vi "Alarms FP FGV.vi"(6 "FP Open in":bool, 7 "Function":enum16{"Read", "Write", "Clear"}(ring)) -> (2 "FP Open out":bool)   [LabVIEW 2020]
panel:
  out "error out":errorcluster
  in  "error in":errorcluster
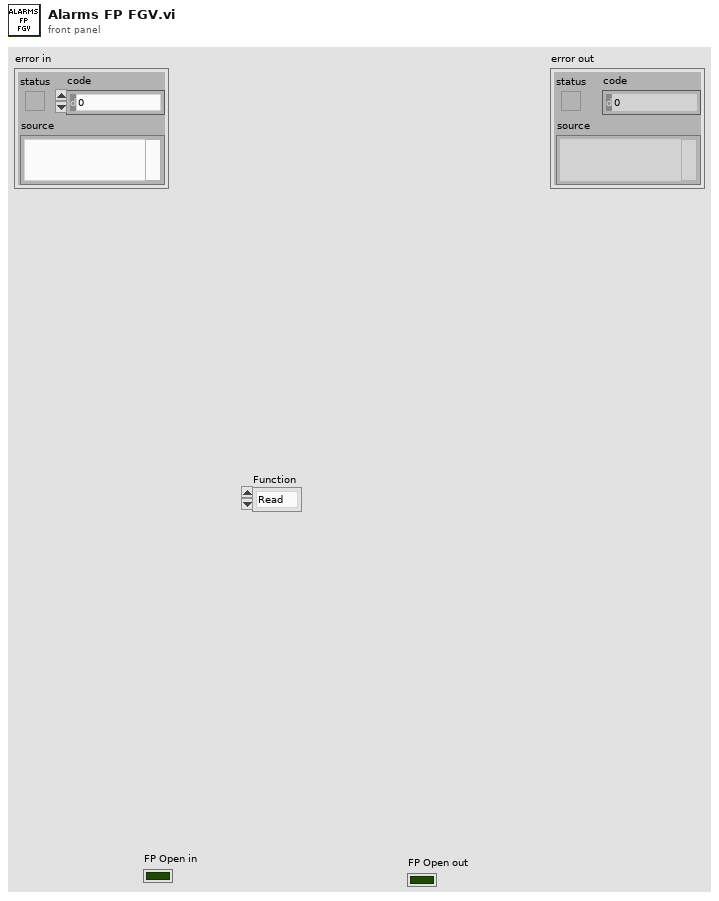
[diagram p1: front panel]
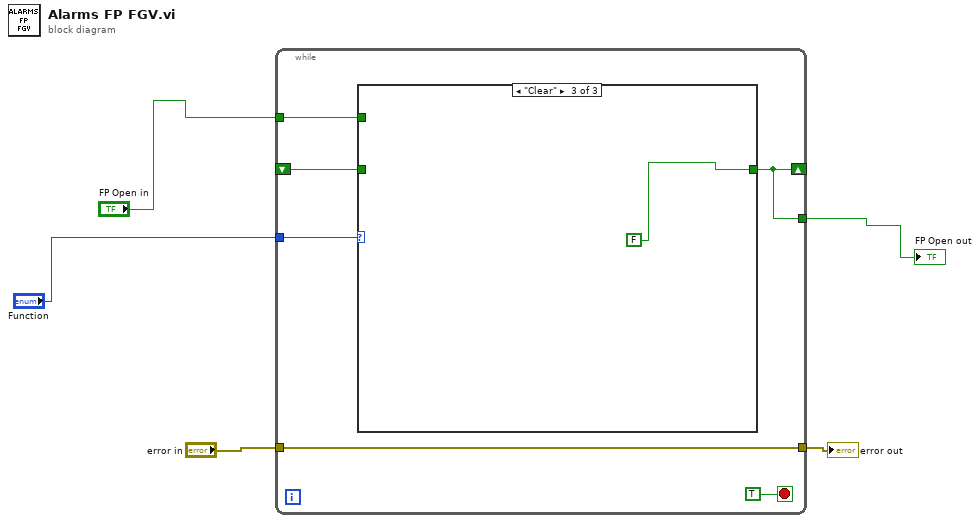
[diagram p0: block diagram]
diagram:
  n1 = while {
    tunnel: "Function" -> [w10]
    shift-right: [w7] -> _
    shift-left: _ -> [w8]
    tunnel: "FP Open in" -> [w9]
    tunnel: [w7] -> w1
    tunnel: "error in" -> [w6]
    tunnel: [w6] -> w3
    stop <- TRUE stop-if-true
    n2 = case shown="\"Clear\"" w10 {
      tunnel: [w12 w13 FALSE ("FP Open out")] -> w7
      tunnel: w9 -> [_ w13 _]
      tunnel: w8 -> [w12 _ _]
      frame "Read", Default {
      }
      frame "Write" {
      }
      frame "Clear" {
      }
    }
  }
  "error out" <- w3
  "FP Open out" <- w1
